vi "ROI entry- Cal Cycles and Acq time final.vi"(4 "number of pixels in miniscan":u16, 6 "<Number of lines>":u16, 9 "Adjust for MC ?":bool, 10 "XYZ_Coordinates":T7[](array[typedef]) {"Apparent Frame Size" format="%#_6f"; "Original FOV (um)" format="%#_6f"; "Pixels per miniscan" format="%#_6f"; "Dwell Time per pixel" format="%#_6f"; "Resolution" format="%#_6f"; "ROI group ID" format="%#_6f"; "Laser Power (%)" format="%#_6f"; "Zoom" format="%#_6f"; "Frame Size" format="%#_6f"; "Number of lines" format="%#_6f"; "Composite ID" format="%#_6f"; "Angle (deg)" format="%#_6f"; "ROI Time (ns)" format="%#_6f"; "ROI ID" format="%#_6f"; "Pixels in ROI" format="%#_6f"; "ROI index" format="%#_6f"; "Z stop" format="%#_6f"; "Y stop" format="%#_6f"; "X stop" format="%#_6f"; "Z start" format="%#_6f"; "X start" format="%#_6f"; "Y start" format="%#_6f"}, 11 "AOL Globals":T1={"Imaging Protocol"=enum."AOL Z-Stack", "Number of POI"=0, "Number of Miniscans"=0, "Number of Trials"=0, "Number of Cycles "=0, "# Averaged Frames"=0, "Laser power (%)"=0, "Pockels (V)"=0.0, "Acquisition Length (sec)"=0.0, "Fill time (us)"=0.0, "POI Dwell time (us)"=0.0, "Miniscan Dwell time per pixel (us)"=0.0, "PMT 1"=0.0, "PMT 2"=0.0, "Back Apperture (mA)"=0.0, "Frame Size"=0, "Center Frequency"=0.0, "Field of View (um)"=175.0, "Field of View (norm)"=0.0, "DwellTime (us)"=0.0, "Ref Dwell Time (us)"=0.0, "Wavelength (nm)"=0.0, "Zoom"=0.0, "AOL Z"=0.0, "AOL Mode"=enum."Raster", "GridXY"=0.0, "GridZ"=0.0, "TriggerPeriod (sec)"=0.0, "Number of Pixels in Miniscan"=0, "Experiment folder path"=path "", "X centre"=0.0, "Y centre"=0.0, "Angle (degrees)"=0.0, "Angle Xs (degrees)"=0.0, "Angle Ys (degrees)"=0.0, "Plane Mode"=0, "Threshold"=[], "Regenerate Chirps"=FALSE, "Rectangle ROI length (pixels)"=0, "Rectangle ROI height (pixels)"=0, "AOD fill"=0, "StartupDelay"=0, "Samples Wait after Trigger"=0, "Slip Cycle"=0, "Add Cycle"=FALSE, "Functional Mode"=enum."Point", "Z Start"=0.0, "Z Stop"=0.0, "# Planes"=0, "Total Pixels"=0, "Variable Miniscan Pixels"=[], "Use Variable Length"=FALSE, "Use Variable Resolution"=FALSE, "Laser power (%) at Z Start"=0, "Laser power (%) at Z Stop"=0, "Ref Z Step"=0} {"Angle Ys (degrees)" format="%#.6g"; "Angle Xs (degrees)" format="%#.6g"; "Plane Mode" items=["XY Plane", "XZ Plane", "YZ Plane", "arbitraryplane"]; "Frame Size" items=["100X100"=100, "128X128"=128, "200X200"=200, "256X256"=256, "512X512"=512, "1024x1024"=1024, "2048x2048"=2048]; "Back Apperture (mA)" format="%#.6g"; "Pockels (V)" format="%#.6g"; "PMT 2" format="%#.6g"; "PMT 1" format="%#.6g"; "Angle (degrees)" format="%#.6g"; "POI Dwell time (us)" format="%#.6g"}) -> (2 "number of cycles":u64, 3 "Acq length":dbl)   [LabVIEW 2020]
uses:
  Visualisation/Functional Imaging Viewer/Typedefs/ROI parameters data type.ctl
  Typedefs/Controls/AOL_Globals.ctl
  Typedefs/Imaging Protocols enum.ctl
  Typedefs/Frame Size.ctl
  Typedefs/AOL modes.ctl
  Typedefs/Plane Mode.ctl
  Typedefs/Functional Mode.ctl
  Global Variables/General Globals.vi
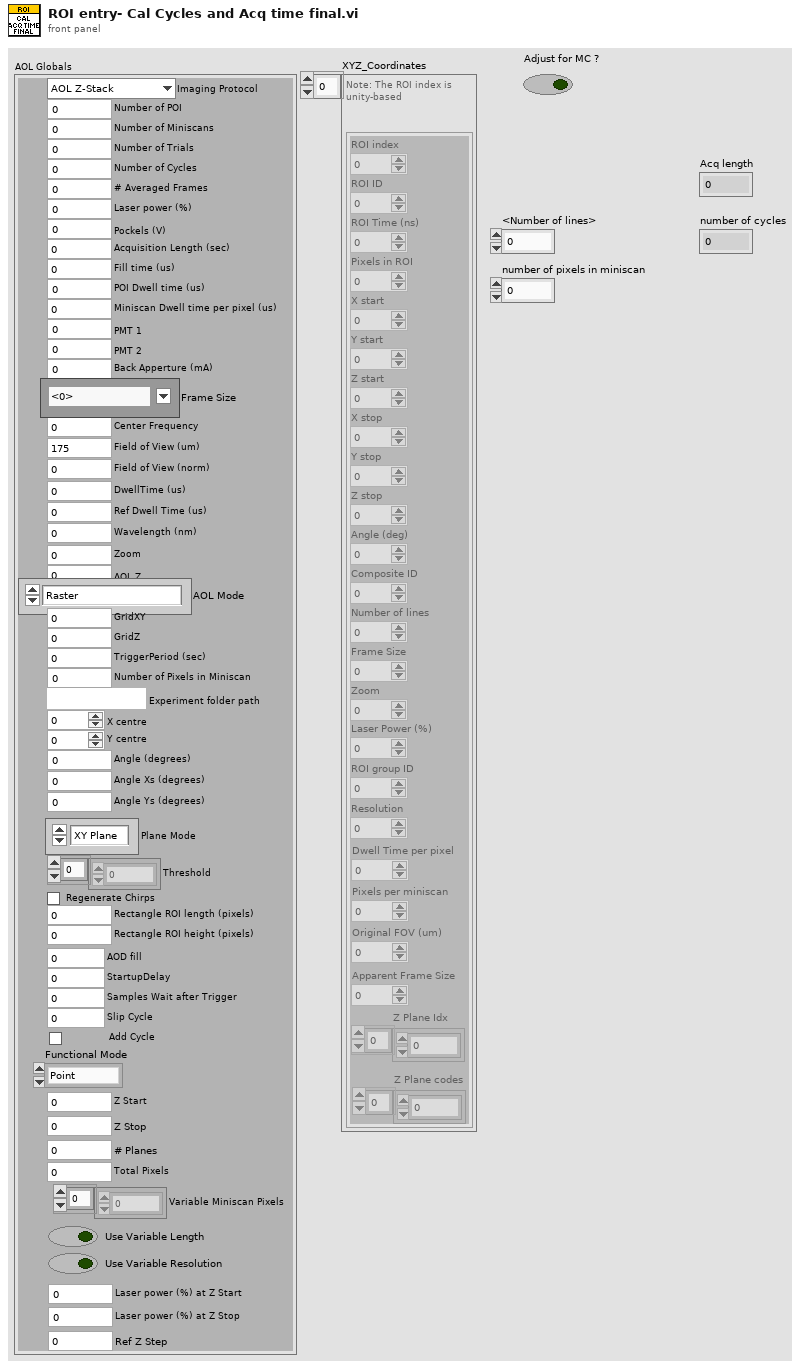
[diagram p1: front panel]
types:
  T1 = typedef "AOL_Globals.ctl" = cluster{"Imaging Protocol":T2, "Number of POI":u16, "Number of Miniscans":u16, "Number of Trials":u16, "Number of Cycles ":u64, "# Averaged Frames":u16, "Laser power (%)":u8, "Pockels (V)":dbl, "Acquisition Length (sec)":dbl, "Fill time (us)":dbl, "POI Dwell time (us)":dbl, "Miniscan Dwell time per pixel (us)":dbl, "PMT 1":dbl, "PMT 2":dbl, "Back Apperture (mA)":dbl, "Frame Size":T3, "Center Frequency":dbl, "Field of View (um)":dbl, "Field of View (norm)":dbl, "DwellTime (us)":dbl, "Ref Dwell Time (us)":dbl, "Wavelength (nm)":dbl, "Zoom":dbl, "AOL Z":dbl, "AOL Mode":T4, "GridXY":dbl, "GridZ":dbl, "TriggerPeriod (sec)":dbl, "Number of Pixels in Miniscan":u16, "Experiment folder path":path, "X centre":dbl, "Y centre":dbl, "Angle (degrees)":dbl, "Angle Xs (degrees)":dbl, "Angle Ys (degrees)":dbl, "Plane Mode":T5, "Threshold":u16[], "Regenerate Chirps":bool, "Rectangle ROI length (pixels)":u16, "Rectangle ROI height (pixels)":u16, "AOD fill":u16, "StartupDelay":i32, "Samples Wait after Trigger":u16, "Slip Cycle":u32, "Add Cycle":bool, "Functional Mode":T6, "Z Start":dbl, "Z Stop":dbl, "# Planes":i32, "Total Pixels":i32, "Variable Miniscan Pixels":u16[], "Use Variable Length":bool, "Use Variable Resolution":bool, "Laser power (%) at Z Start":u8, "Laser power (%) at Z Stop":u8, "Ref Z Step":i8}
  T2 = typedef "Imaging Protocols enum.ctl" = enum16{"AOL Z-Stack", "Motor Z Stack", "Parameter Sweep", "Functional Acquisition", "Single Plane Acquisition", "Volume Acquisition", "Live Imaging", "Live Plane Imaging", "Live Volume Imaging"}
  T3 = typedef "Frame Size.ctl" = u16
  T4 = typedef "AOL modes.ctl" = enum16{"Raster", "Structural", "Pointing", "Mini Scan", "Alignment"}
  T5 = typedef "Plane Mode.ctl" = u16
  T6 = typedef "Functional Mode.ctl" = enum16{"Point", "Line", "Patch", "Plane", "Volume"}
  T7 = typedef "ROI parameters data type.ctl" = cluster{"ROI index":dbl, "ROI ID":dbl, "ROI Time (ns)":dbl, "Pixels in ROI":dbl, "X start":dbl, "Y start":dbl, "Z start":dbl, "X stop":dbl, "Y stop":dbl, "Z stop":dbl, "Angle (deg)":dbl, "Composite ID":dbl, "Number of lines":dbl, "Frame Size":dbl, "Zoom":dbl, "Laser Power (%)":dbl, "ROI group ID":dbl, "Resolution":dbl, "Dwell Time per pixel":dbl, "Pixels per miniscan":dbl, "Original FOV (um)":dbl, "Apparent Frame Size":dbl, "Z Plane Idx":i32[], "Z Plane codes":i32[]}
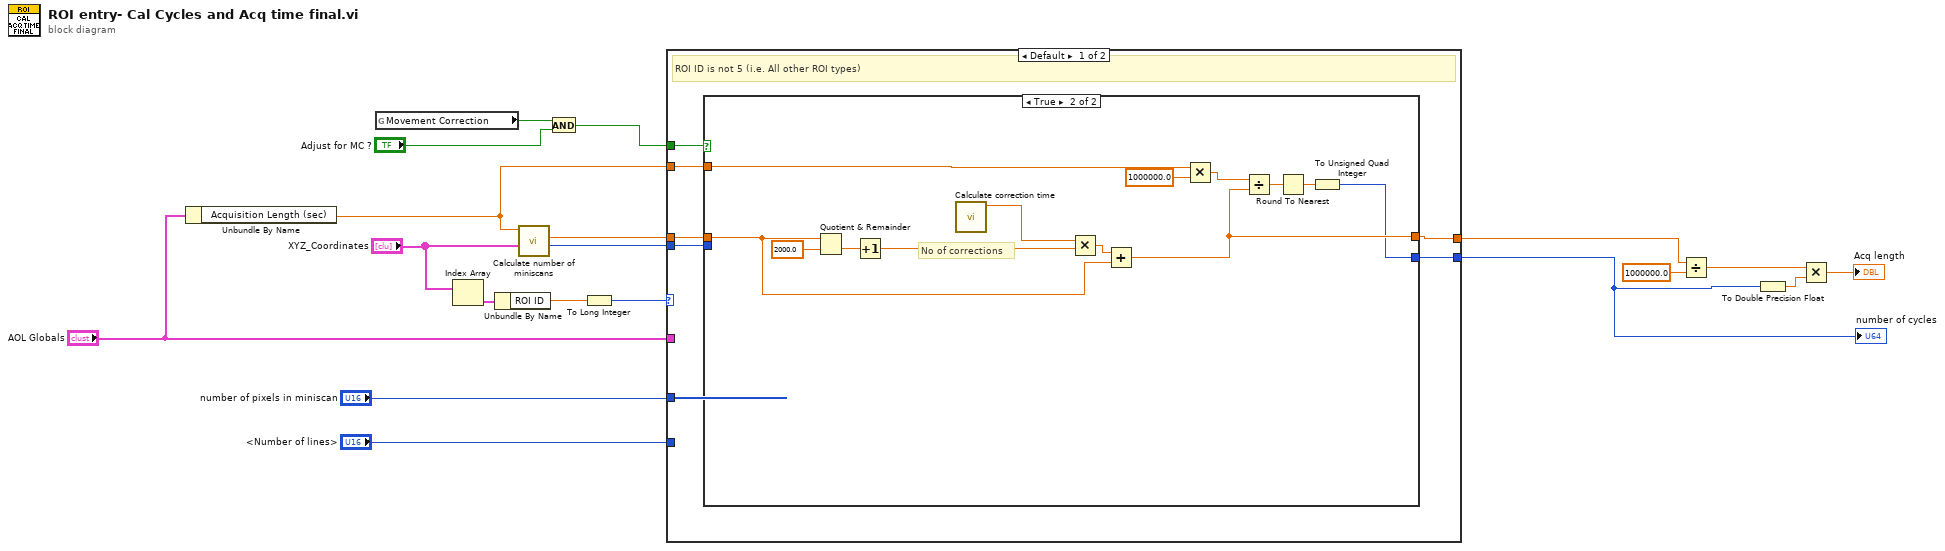
[diagram p0: block diagram]
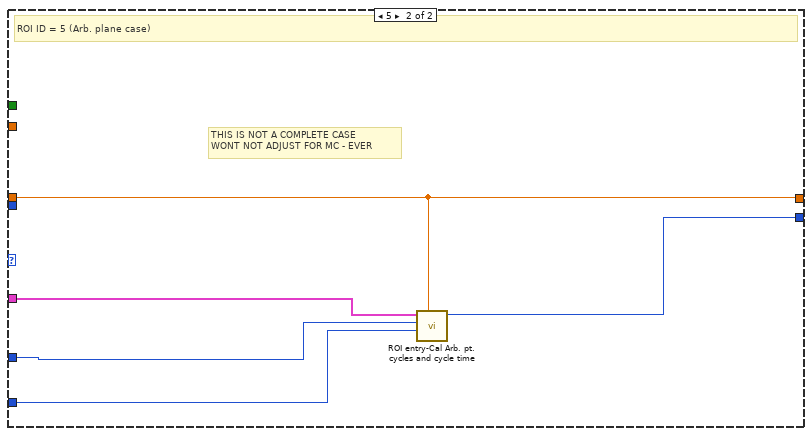
[diagram p3: hidden frame]
diagram:
  n1 = Unbundle By Name("AOL Globals") -> ("Acquisition Length (sec)"=w4:dbl)
  n2 = global read "General Globals.vi" "Movement Correction"() -> (w3:bool)
  n3 = Index Array(array="XYZ_Coordinates") -> (element=w10:T7)  [unwired: 1 in]
  n4 = Unbundle By Name(w10) -> ("ROI ID"=w11:dbl)
  n5 = call "Calculate number of miniscans.vi"("XYZ Coordinates"="XYZ_Coordinates", "Acquisition length (sec)"=w4) -> ("Number of cycles"=w7:u64, "Cycle time (us)"=w8:dbl)  [unwired: 7 in, 1 out]
  n6 = And(x=w3, y="Adjust for MC ?") -> (x .and. y?=w1:bool)
  n7 = To Long Integer(number=w11) -> (32bit integer=w12:i32)
  n8 = case shown="Default" w12 {
    tunnel: "number of pixels in miniscan" -> [_ w45]
    tunnel: "<Number of lines>" -> [_ w44]
    tunnel: "AOL Globals" -> [_ w43]
    tunnel: [w22 w42] -> w16
    tunnel: w1 -> [w25 _]
    tunnel: w8 -> [w24 w41]
    tunnel: w7 -> [w23 _]
    tunnel: [w21 w41] -> w6
    tunnel: w4 -> [w20 _]
    frame Default {
      # "ROI ID is not 5 (i.e. All other ROI types)"
      n9 = case shown="True" w25 {
        tunnel: w24 -> [w26 w35]
        tunnel: w23 -> [w27 _]
        tunnel: [w27 w28] -> w22
        tunnel: [w26 w31] -> w21
        tunnel: w20 -> [_ w34]
        frame False {
        }
        frame True {
          # "No of corrections"
          n10 = Quotient & Remainder(x=w35, y=2000.0) -> (floor(x/y)=w39:dbl)  [unwired: 1 out]
          n11 = Increment(x=w39) -> (x+1=w38:dbl)
          n12 = call "Calculate correction time.vi"() -> ("Correction time"=w37:dbl)  [unwired: 11 in]
          n13 = Multiply(x=w37, y=w38) -> (x*y=w36:dbl)
          n14 = Add(x=w36, y=w35) -> (x+y=w31:dbl)
          n15 = Multiply(x=w34, y=1000000.0) -> (x*y=w32:dbl)
          n16 = Divide(x=w32, y=w31) -> (x/y=w29:dbl)
          n17 = Round To Nearest(number=w29) -> (nearest integer value=w30:dbl)
          n18 = To Unsigned Quad Integer(1:w30) -> (0:w28:u64)
        }
      }
    }
    frame 5 {
      # "THIS IS NOT A COMPLETE CASE\nWONT NOT ADJUST FOR MC - EVER"
      # "ROI ID = 5 (Arb. plane case)"
      n19 = call "ROI entry-Cal Arb. pt. cycles and cycle time.vi"("Cycle time"=w41, "<Number of lines>"=w44, "number of pixels in miniscan"=w45, "AOL Globals"=w43) -> ("No lof cycles"=w42:u64)  [unwired: 7 in]
    }
  }
  "number of cycles" <- w16
  n20 = Divide(x=w6, y=1000000.0) -> (x/y=w15:dbl)
  n21 = To Double Precision Float(number=w16) -> (double precision float=w17:dbl)
  n22 = Multiply(x=w15, y=w17) -> (x*y=→"Acq length":dbl)
